vi "massflow.vi"() -> ()   [LabVIEW 2023]
uses:
  <vilib>/Waveform/WDTOps.llb/WDT Append Waveforms DBL.vi
  <vilib>/Waveform/WDTFileIO.llb/Export Waveform To Spreadsheet File.vi
panel:
  in  "stop":bool
  in  "Flow full scale":dbl
  out "Waveform Chart":dynamicdata(graph)
  out "Flow(cubic cm)":dbl
  out "% Full Scale":dbl
  out "voltage":dbl
  in  "Setpoint":dbl
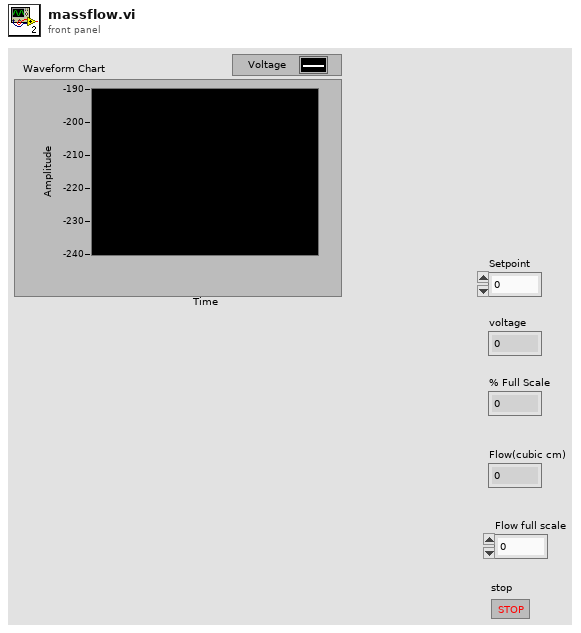
[diagram p1: front panel]
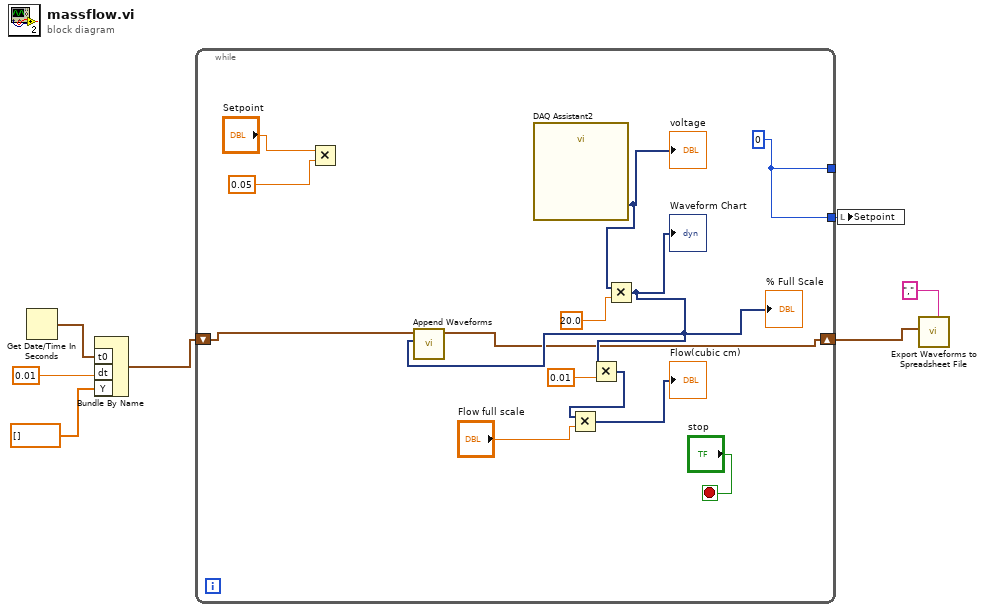
[diagram p0: block diagram]
diagram:
  n1 = Get Date/Time In Seconds() -> (seconds since 1Jan1904=w4:timestamp)
  n2 = Bundle By Name("t0"=w4, "dt"=0.01, "Y"=dbl[] []) -> (w3:waveform(dbl))  [unwired: 1 in]
  n3 = while {
    tunnel: [w11] -> _
    tunnel: [w11] -> w7
    shift-right: [w8] -> w2
    shift-left: w3 -> [w10]
    stop <- "stop" stop-if-true
    w11 = 0
    n4 = Multiply(x="Setpoint", y=0.05) -> ()  [unwired: 1 out]
    n5 = call "DAQ Assistant2"() -> ("data"=w18:dynamicdata)  [unwired: 16 in, 3 out]
    "voltage" <- w18
    n6 = Multiply(x=w18, y=20.0) -> (x*y=w9:dynamicdata)
    "% Full Scale" <- w9
    "Waveform Chart" <- w9
    n7 = call-poly <vilib>:"Append Waveforms.vi"("waveform B"=w9, "waveform A"=w10) -> ("waveform out"=w8:waveform(dbl))  [unwired: 8 in, 1 out]
    n8 = Multiply(x=w9, y=0.01) -> (x*y=w15:dynamicdata)
    n9 = Multiply(x=w15, y="Flow full scale") -> (x*y=→"Flow(cubic cm)":dynamicdata)
  }
  n10 = local write "Setpoint"(w7) -> ()
  n11 = call-poly <vilib>:"Export Waveforms to Spreadsheet File.vi"("delimiter (Tab)"=",", "waveform"=w2) -> ()  [unwired: 8 in, 2 out]
